vi "autoMain.vi"() -> ()   [LabVIEW 2012]
uses:
  <vilib>/Platform/TimedLoop/XDataNode/nitl_modes.ctl
  <vilib>/Platform/TimedLoop/XDataNode/timing_clust.ctl
  <vilib>/Platform/TimedLoop/XDataNode/wakeup.ctl
  <vilib>/platform/TimedLoop/XDataNode/XDataNode.xnode
  <vilib>/Platform/TimedLoop/XDataNode/XDNodeRunTimeDep.lvlib
  <vilib>/Rock Robotics/SystemInterfaces/AI/FPGA_AIGyroChannel.ctl
panel:
  out "sensor datas":T1
  out "Time between Iterations":u32
  out "Elapsed Auto Time":dbl
  out "Numeric 3":i32
  out "Numeric 2":i32
  out "Numeric":i32
  out "commands from file":string[][](array[string])
  out "Active Commands":string[][](array[string])
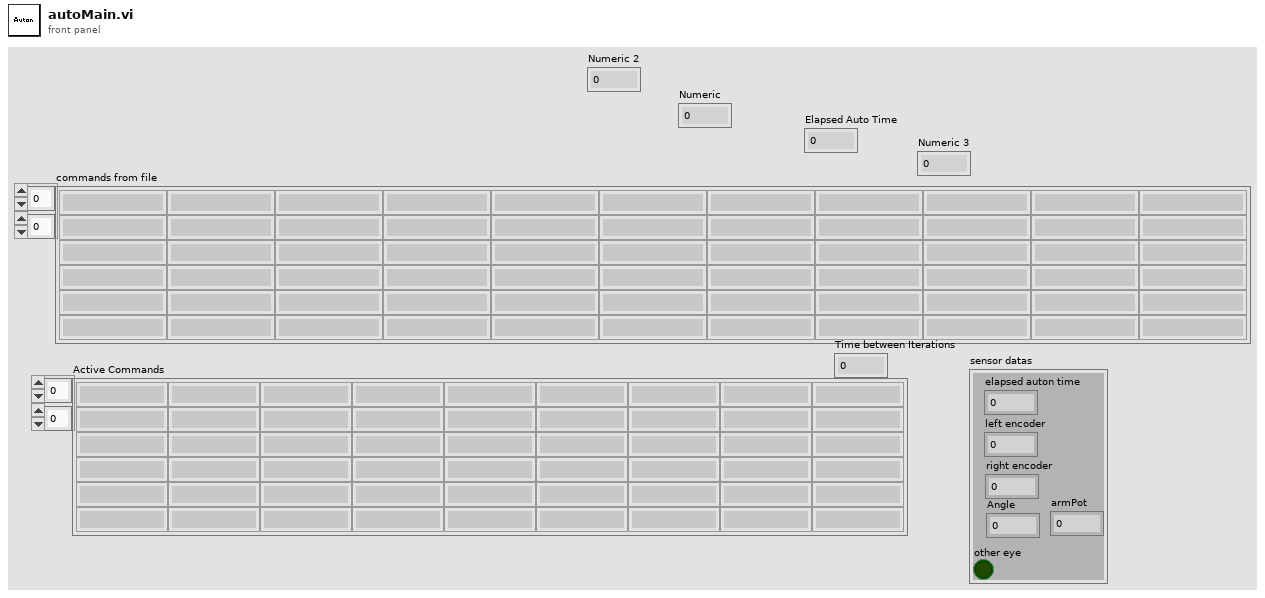
[diagram p1: front panel]
types:
  T1 = cluster{"elapsed auton time":dbl, "left encoder":dbl, "other eye":bool, "right encoder":dbl, "Angle":dbl, "armPot":dbl}
  T2 = typedef "XDNodeRunTimeDep.lvlib/nitl_modes.ctl" = enum32{"No Change", "Process missed periods, maintain original phase", "Discard missed periods, maintain original phase", "Process missed periods, ignore original phase", "Discard missed periods, ignore original phase"}
  T3 = typedef "FPGA_AIGyroChannel.ctl" = enum8{"AI 1", "AI 2", "Invalid"}
  T4 = typedef "WPI_GyroDevRef.ctl" = cluster{"DevStatus":errorcluster, "Analog Module":T5, "Analog Channel":T6, "Offset":dbl, "Gain (VoltsPerDegree/Second)":dbl}
  T5 = typedef "FPGA_TypedefAnalogModule.ctl" = enum16{"Analog Module 1", "Analog Module 2"}
  T6 = typedef "FPGA_AIChannel.ctl" = enum8{"AI 1", "AI 2", "AI 3", "AI 4", "AI 5", "AI 6", "AI 7", "AI 8", "Invalid"}
  T7 = typedef "XDNodeRunTimeDep.lvlib/timing_clust.ctl" = cluster{"Expected End [f-1]":u64, "Actual End [f-1]":u64, "Finished Late? [f-1]":bool, "Expected End [i-1]":u64, "Actual End [i-1]":u64, "Finished Late? [i-1]":bool, "Expected Start [i]":u64, "Actual Start [i]":u64, "Expected Start [f]":u64, "Actual Start [f]":u64, "Source Name":string, "Structure Name":string, "Period":i64, "Deadline":i64, "Offset":i64, "Start":i64, "Priority":i32, "Timeout":i32, "Mode":T2, "Wakeup Reason":T8, "Error":errorcluster, "Source Type":string, "Secondary Source Type":string, "Global End Time":u64, "Global Start Time":u64, "Frame Duration":u64, "Iteration Duration":u64, "Assigned CPU":i32, "I/O Scan Engine Mode":u32}
  T8 = typedef "XDNodeRunTimeDep.lvlib/wakeup.ctl" = enum32{"Normal", "Aborted", "Asynchronous wakeup", "Timing source error", "Timed loop error", "Timeout"}
  T9 = cluster{"elapsed auton time":dbl, "left encoder":dbl, "other eye":bool, "right encoder":dbl, "Angle":dbl, "Angle 2":dbl}
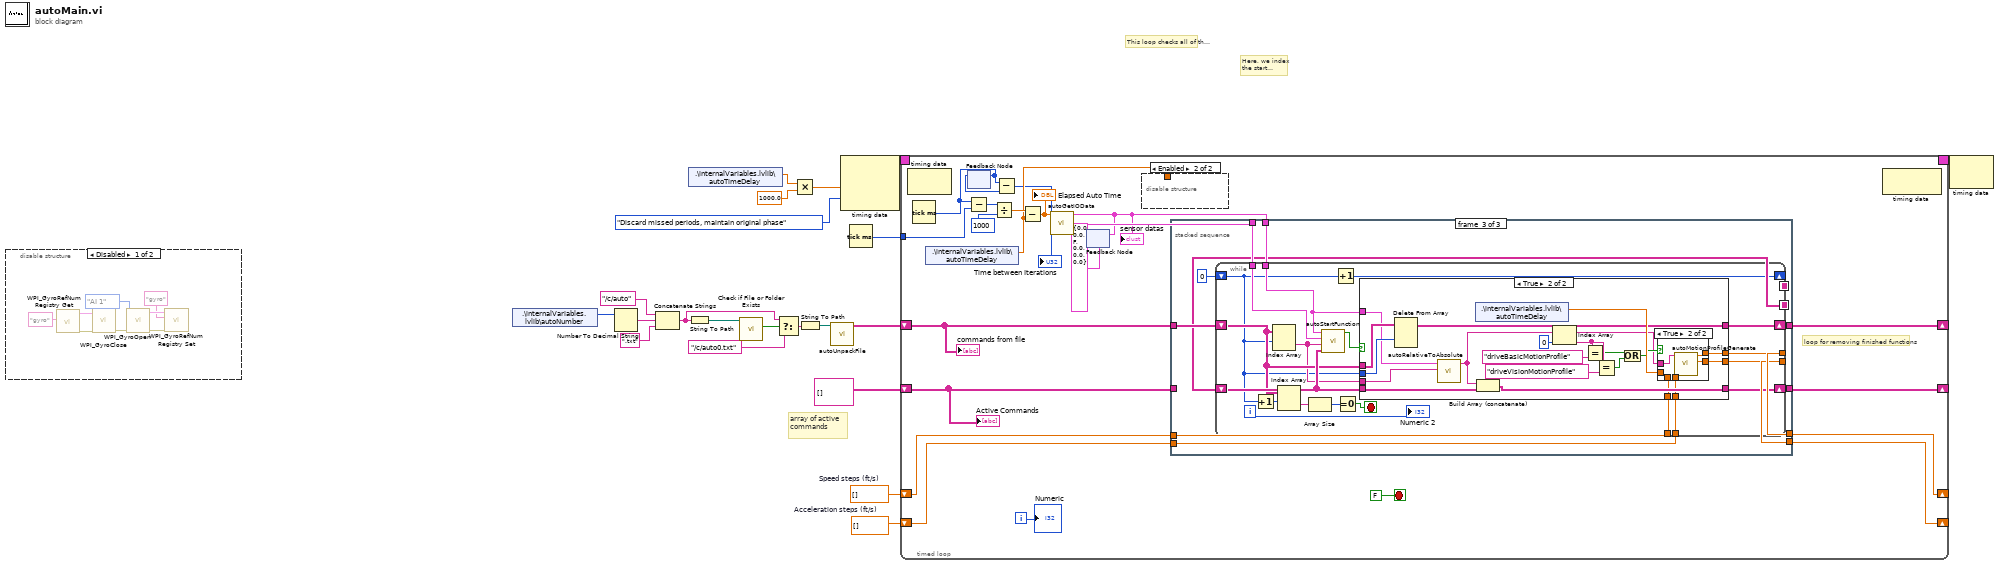
[diagram p0: block diagram]
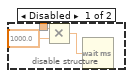
[diagram p3: hidden frame]
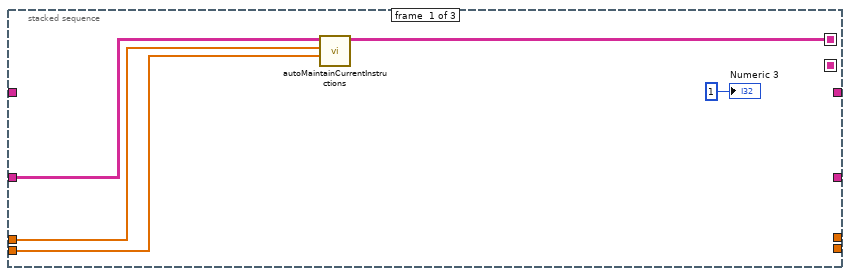
[diagram p4: hidden frame]
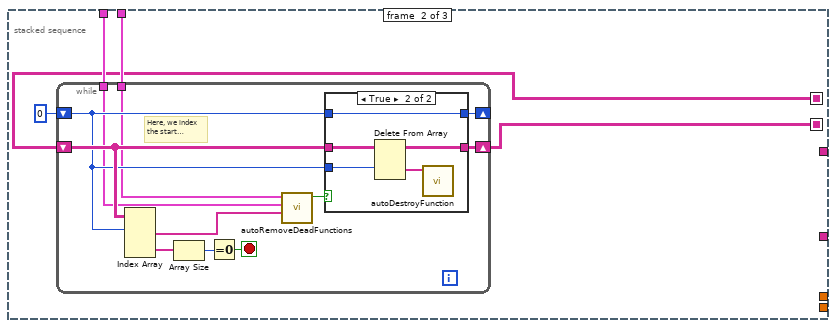
[diagram p5: hidden frame]
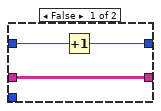
[diagram p6: hidden frame]
diagram:
  w15 = dbl[] []  # Acceleration steps (ft/s)
  w16 = dbl[] []  # Speed steps (ft/s)
  # "array of active commands"
  # "This loop checks all of the commands in the command/parameter array and adds the appropiate ones to the list of commands currently being executed."
  # "Here, we index the start condition type and value."
  n1 = disable-structure shown="Disabled" {
    frame Disabled {
      n2 = call <vilib>:"WPI_GyroRefNum Registry Get.vi"("refnum name"="gyro") -> ("error out"=w29:errorcluster, "GyroDevRef"=w28:T4)  [unwired: 9 in]
      n3 = call <vilib>:"WPI_GyroClose.vi"("error in (no error)"=w29, "GyroDevRef"=w28) -> ("error out"=w27:errorcluster)  [unwired: 9 in]
      n4 = call <vilib>:"WPI_GyroOpen.vi"("error in (no error)"=w27, "Analog Channel"=FPGA_AIGyroChannel."AI 1") -> ("error out"=w26:errorcluster, "GyroDevRef"=w25:T4)  [unwired: 7 in, 1 out]
      n5 = call <vilib>:"WPI_GyroRefNum Registry Set.vi"("error in (no error)"=w26, "refnum name"="gyro", "GyroDevRef"=w25) -> ()  [unwired: 7 in, 2 out]
    }
    frame Enabled {
    }
  }
  n6 = shared-variable ".\\internalVariables.lvlib\\autoNumber"() -> (w1:i16)  [unwired: 1 in, 1 out]
  n7 = Number To Decimal String(number=w1) -> (decimal integer string=w8:string)  [unwired: 1 in]
  n8 = Concatenate Strings("/c/auto", w8, ".txt" ("string")) -> (w4:string)
  n9 = String To Path(string=w4) -> (path=w6:path)
  n10 = shared-variable ".\\internalVariables.lvlib\\autoTimeDelay"() -> (w14:dbl)  [unwired: 1 in, 1 out]
  n11 = call <vilib>:"Check if File or Folder Exists.vi"("path"=w6) -> ("file or folder exists?"=w5:bool)  [unwired: 8 in, 2 out]
  n12 = Select(t=w4, s=w5, f="/c/auto0.txt") -> (s? t:f=w2:string)
  n13 = Multiply(x=w14, y=1000.0) -> (x*y=w11:dbl)
  n14 = String To Path(string=w2) -> (path=w10:path)
  n15 = call "autoUnpackFile.vi"("file path in"=w10) -> ("command/parameter array out"=w18:string[][])  [unwired: 10 in]
  n16 = node-c288(w11, nitl_modes."Discard missed periods, maintain original phase" ("Mode")) -> (w21:T7)  [unwired: 1 in]
  n17 = Tick Count (ms)() -> (millisecond timer value=w17:u32)
  n18 = timed-loop {
    shift-right: [w41] -> _
    shift-left: string[][] [] -> [w51]
    shift-right: [w42] -> _
    shift-left: w18 -> [w50]
    tunnel: w17 -> [w32]
    shift-right: [w38] -> _
    shift-left: w16 -> [w30]
    shift-right: [w36] -> _
    shift-left: w15 -> [w37]
    timing: w21 -> [_]
    timing-out: [_] -> w20
    i -> [w48]
    stop <- FALSE stop-if-true
    # "loop for removing finished functions"
    n19 = node-c288() -> ()  [unwired: 1 in, 1 out]
    n20 = Tick Count (ms)() -> (millisecond timer value=w35:u32)
    n21 = shared-variable ".\\internalVariables.lvlib\\autoTimeDelay"() -> (w33:dbl)  [unwired: 1 in, 1 out]
    n22 = feedback-in #1(w35) -> ()
    n23 = feedback #1() -> (w34:u32)  [unwired: 1 in]
    n24 = Subtract(x=w35, y=w32) -> (x-y=w47:u32)
    n25 = Divide(x=w47, y=u32 1000) -> (x/y=w43:dbl)
    n26 = Subtract(x=w35, y=w34) -> (x-y=→"Time between Iterations":u32)
    n27 = Subtract(x=w43, y=w33) -> (x-y=w44:dbl)
    "Elapsed Auto Time" <- w44
    n28 = call "autoGetIOData.vi"("elapsed auton time"=w44) -> ("sensor datas"=w39:T1)  [unwired: 10 in]
    "sensor datas" <- w39
    n29 = feedback #2(T9 {"elapsed auton time"=0.0, "left encoder"=0.0, "other eye"=FALSE, "right encoder"=0.0, "Angle"=0.0, "Angle 2"=0.0} ("const")) -> (w45:T9)
    n30 = feedback-in #2(w39) -> ()
    n31 = disable-structure shown="Enabled" {
      disable-tunnel: w33 -> [w53 _]
      frame Disabled {
        n32 = Multiply(x=w53, y=1000.0) -> (x*y=w52:dbl)
        n33 = Wait (ms)(milliseconds to wait=w52) -> ()  [unwired: 1 out]
      }
      frame Enabled {
      }
    }
    n34 = stacked-sequence {
      seq-local: [_ w63 _] -> [_ _ w90]
      seq-local: [w61 _ _] -> [_ w62 _]
      tunnel: w51 -> [w60 _ _]
      tunnel: w50 -> [_ _ w93]
      tunnel: w39 -> [_ w64 w96]
      tunnel: w45 -> [_ w65 w95]
      tunnel: [_ _ w92] -> w42
      tunnel: [_ _ w91] -> w41
      tunnel: w30 -> [w57 _ w88]
      tunnel: [_ _ w89] -> w38
      tunnel: w37 -> [w59 _ w86]
      tunnel: [_ _ w87] -> w36
      frame #0 {
        n35 = call "autoMaintainCurrentInstructions.vi"("MotionProfile acceleration"=w59, "MotionProfile speed"=w57, "running commands"=w60) -> ("running commands out"=w61:string[][])  [unwired: 5 in, 1 out]
        "Numeric 3" <- 1 ("Numeric 3")
      }
      frame #1 {
        n36 = while {
          shift-right: [w76] -> w63
          shift-left: w62 -> [w77]
          shift-right: [w74] -> _
          shift-left: 0 -> [w73]
          tunnel: w65 -> [w70]
          tunnel: w64 -> [w69]
          stop <- w71 stop-if-true
          # "Here, we index the start condition type and value."
          n37 = Index Array(array=w77, index (row) #1=w73) -> (element #1=w68:string[], element #2=w67:string[])  [unwired: 3 in]
          n38 = Array Size(array=w67) -> (size(s)=w72:i32)
          n39 = Equal To 0?(x=w72) -> (x = 0?=w71:bool)
          n40 = call "autoRemoveDeadFunctions.vi"("command in"=w68, "old sensor datas"=w70, "sensor datas"=w69) -> ("remove"=w75:bool)  [unwired: 8 in]
          n41 = case shown="True" w75 {
            tunnel: [w80 w84] -> w76
            tunnel: w77 -> [w80 w85]
            tunnel: w73 -> [_ w83]
            tunnel: w73 -> [w79 w81]
            tunnel: [w78 w81] -> w74
            frame False {
              n42 = Increment(x=w79) -> (x+1=w78:i32)
            }
            frame True {
              n43 = Delete From Array(array=w85, index (row)=w83) -> (deleted portion=w82:string[], array with subset deleted=w84:string[][])  [unwired: 2 in]
              n44 = call "autoDestroyFunction.vi"("command in"=w82) -> ()  [unwired: 11 in]
            }
          }
        }
      }
      frame #2 {
        n45 = while {
          shift-right: [w114] -> w91
          shift-left: w90 -> [w112]
          shift-right: [w113] -> w92
          shift-left: w93 -> [w108]
          tunnel: w96 -> [w110]
          tunnel: w95 -> [w111]
          shift-right: [w100] -> _
          shift-left: 0 -> [w99]
          tunnel: [w102] -> w89
          tunnel: w88 -> [w101]
          tunnel: [w98] -> w87
          tunnel: w86 -> [w97]
          i -> [w104]
          stop <- w105 stop-if-true
          n46 = Increment(x=w99) -> (x+1=w109:i32)
          n47 = Index Array(array=w108, index (row)=w99) -> (element=w103:string[])  [unwired: 1 in]
          n48 = Index Array(array=w108, index (row)=w109) -> (element=w107:string[])  [unwired: 1 in]
          n49 = Array Size(array=w107) -> (size(s)=w106:i32)
          n50 = call "autoStartFunction.vi"("running command array"=w112, "command in"=w103, "old sensor datas"=w111, "sensor datas"=w110) -> ("start?"=w115:bool)  [unwired: 7 in]
          n51 = Increment(x=w99) -> (x+1=w100:i32)
          n52 = Equal To 0?(x=w106) -> (x = 0?=w105:bool)
          n53 = case shown="True" w115 {
            tunnel: [w116 w131] -> w113
            tunnel: w112 -> [w119 w137]
            tunnel: w103 -> [_ w135]
            tunnel: w108 -> [w116 w139]
            tunnel: w99 -> [_ w138]
            tunnel: [w119 w136] -> w114
            tunnel: w110 -> [_ w134]
            tunnel: [w118 w133] -> w102
            tunnel: w101 -> [w118 w123]
            tunnel: [w117 w121] -> w98
            tunnel: w97 -> [w117 w120]
            frame False {
            }
            frame True {
              n54 = Delete From Array(array=w139, index (row)=w138) -> (array with subset deleted=w131:string[][])  [unwired: 2 in, 1 out]
              n55 = call "autoRelativeToAbsolute.vi"("command in"=w135, "datas"=w134) -> ("adjusted command"=w122:string[])  [unwired: 9 in]
              n56 = shared-variable ".\\internalVariables.lvlib\\autoTimeDelay"() -> (w132:dbl)  [unwired: 1 in, 1 out]
              n57 = Build Array (concatenate)(w122, w137) -> (w136:string[][])
              n58 = Index Array(array=w122, index=0) -> (element=w128:string)
              n59 = Equal?(x=w128, y="driveBasicMotionProfile") -> (x = y?=w125:bool)
              n60 = Equal?(x=w128, y="driveVisionMotionProfile") -> (x = y?=w126:bool)
              n61 = Or(x=w125, y=w126) -> (x .or. y?=w124:bool)
              n62 = case shown="True" w124 {
                tunnel: [w141 w144] -> w133
                tunnel: w132 -> [_ _]
                tunnel: w123 -> [w141 _]
                tunnel: w122 -> [_ w143]
                tunnel: [w140 w142] -> w121
                tunnel: w120 -> [w140 _]
                frame False {
                }
                frame True {
                  n63 = call "autoMotionProfileGenerate.vi"("InputCommand"=w143) -> ("Acceleration steps (ft/s^2)"=w142:dbl[], "Speed steps (ft/s)"=w144:dbl[])  [unwired: 9 in]
                }
              }
            }
          }
          "Numeric 2" <- w104
        }
      }
    }
    n64 = node-c288() -> ()  [unwired: 1 in, 1 out]
    "Active Commands" <- w51
    "commands from file" <- w50
    "Numeric" <- w48
  }
  n65 = node-c288(w20) -> ()  [unwired: 1 out]
